vi "testVector.vi"() -> ()   [LabVIEW 2014]
panel:
  in  "Path 2":path
  in  "Color":u32
  out "output cluster":T1
  out "Division Colors":u32[](array[colorbox])=[16711680, 6618880, 3381759, 16318208]
  out "Pie Chart":picture
  in  "Boolean":bool
  in  "Pie Chart Size (200 pixels)":dbl=200.0
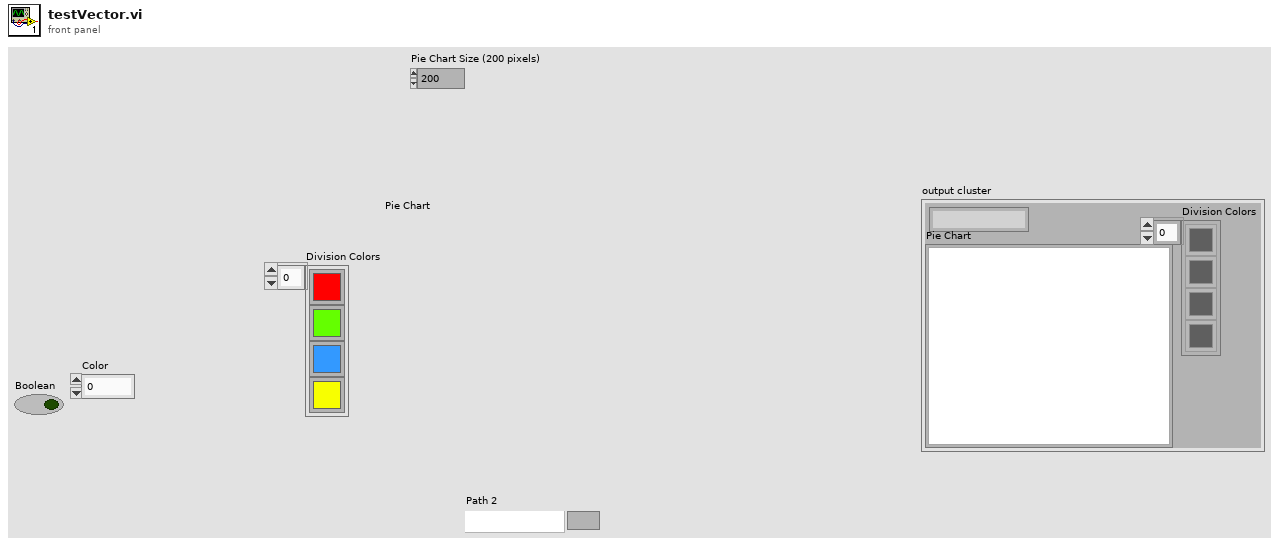
[diagram p1: front panel]
types:
  T1 = cluster{"Division Colors":u32[], "Pie Chart":picture, string}
  T2 = typedef "imagedata.ctl" = cluster{"image type":i32, "image depth":i32, "image":u8[], "mask":u8[], "colors":u32[], "Rectangle":cluster{"left":i16, "top":i16, "right":i16, "bottom":i16}}
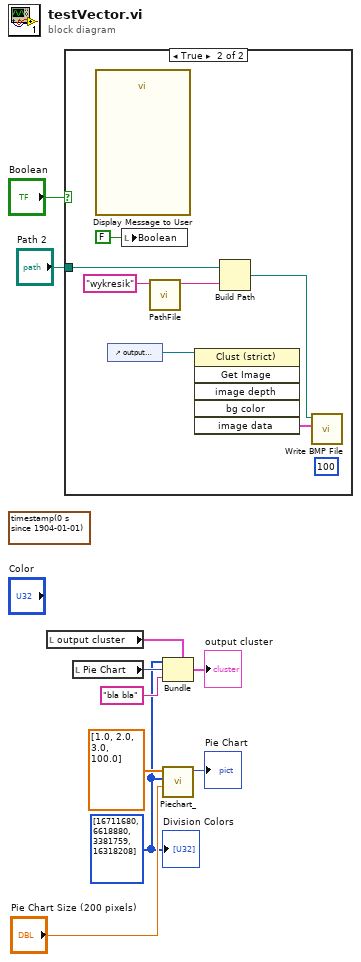
[diagram p0: block diagram]
diagram:
  (unwired) timestamp(0 s since 1904-01-01)
  w2 = u32[] [16711680, 6618880, 3381759, 16318208] ("Division Colors")
  n1 = local read "output cluster"() -> (w4:T1)
  n2 = case shown="True" "Boolean" {
    tunnel: "Path 2" -> [_ w15]
    frame False {
    }
    frame True {
      (unwired) 100 ("quality (80)")
      n3 = call "Display Message to User"() -> ()  [unwired: 10 in, 2 out]
      n4 = control-ref of="output cluster"() -> (w17:refnum<vi>)
      n5 = local write "Boolean"(FALSE) -> ()
      n6 = call "PathFile.vi"("NameFile"="wykresik") -> ("stringNameFile"=w14:string)  [unwired: 10 in]
      n7 = invoke class="Clust (strict)" method="Get Image"(reference=w17) -> ("image data"=w12:T2)  [unwired: 5 in, 5 out]
      n8 = Build Path(base path=w15, name or relative path=w14) -> (appended path=w11:path)
      n9 = call <vilib>:"Write BMP File.vi"("image data"=w12, "path to BMP file"=w11) -> ()  [unwired: 8 in, 2 out]
    }
  }
  n10 = local read "Pie Chart"() -> (w3:picture)
  n11 = Bundle(cluster=w4, "Division Colors"=w2, "Pie Chart"=w3, "bla bla") -> (→"output cluster":T1)
  n12 = call "Piechart_.vi"("Pie Chart Size (200 pixels)"="Pie Chart Size (200 pixels)", "Division Colors"=w2, "Pie Chart Data (arb unit)"=dbl[] [1.0, 2.0, 3.0, 100.0]) -> ("Pie Chart"=→"Pie Chart":picture)  [unwired: 8 in]
  "Division Colors" <- w2
